vi "Simple RT Add-test_harness.vi"(11 "test case ID":string) -> (3 "result":bool)   [LabVIEW 2018]
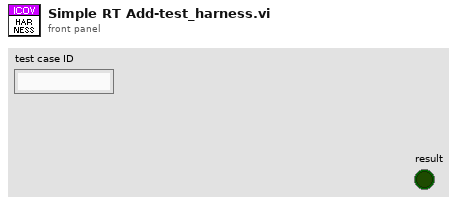
[diagram p1: front panel]
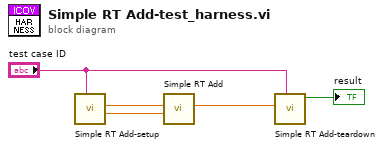
[diagram p0: block diagram]
diagram:
  n1 = call "Simple RT Add-setup.vi"("test case ID"="test case ID") -> ("y"=w3:dbl, "x"=w4:dbl)  [unwired: 9 in]
  n2 = call "Simple RT Add.vi"("y"=w3, "x"=w4) -> ("x+y"=w2:dbl)  [unwired: 8 in, 1 out]
  n3 = call "Simple RT Add-teardown.vi"("test case ID"="test case ID", "Actual x + y result"=w2) -> ("result"=→"result":bool)  [unwired: 9 in]
